vi "setLevel.vi"(0 "VISA resource name 2":refnum<visa-resource-name>, 1 "Source":T1, 2 "Channel":T2, 3 "error out 2":errorcluster, 4 "SourceLevel":dbl) -> (5 "VISA resource name":refnum<visa-resource-name>, 6 "String":string, 7 "error out":errorcluster)   [LabVIEW 2017]
uses:
  controls/Channel.ctl
  controls/Source.ctl
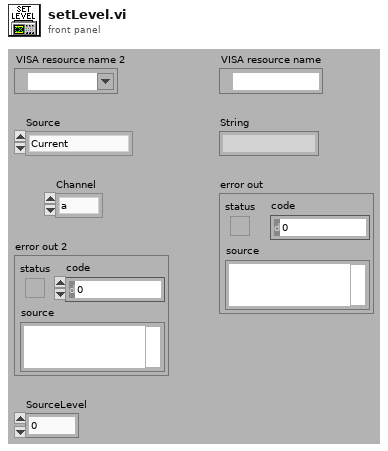
[diagram p1: front panel]
types:
  T1 = typedef "Source.ctl" = enum16{"Current", "Voltage"}
  T2 = typedef "Channel.ctl" = enum16{"a", "b"}
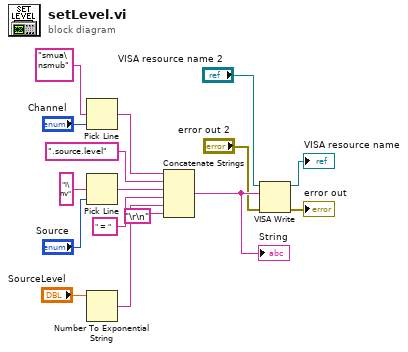
[diagram p0: block diagram]
diagram:
  n1 = Pick Line(multi-line string="smua\nsmub", line index="Channel") -> (output string=w4:string)  [unwired: 1 in]
  n2 = Pick Line(multi-line string="i\nv", line index="Source") -> (output string=w9:string)  [unwired: 1 in]
  n3 = Number To Exponential String(number="SourceLevel") -> (E-format string=w11:string)  [unwired: 3 in]
  n4 = Concatenate Strings(w4, ".source.level", w9, " = " ("string"), w11, "\r\n") -> (w13:string)
  "String" <- w13
  n5 = VISA Write(VISA resource name="VISA resource name 2", write buffer=w13, error in (no error)="error out 2") -> (VISA resource name out=→"VISA resource name":refnum<visa-resource-name>, error out=→"error out":errorcluster)  [unwired: 1 out]
